vi "IntToBoolean.vi"(1 "Input Int":u8[](array[numeric])) -> (0 "Output Boolean":bool[](array[boolean]))   [LabVIEW 2013]
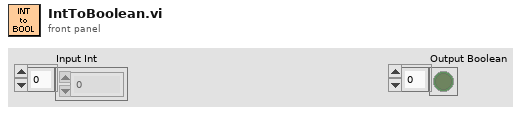
[diagram p1: front panel]
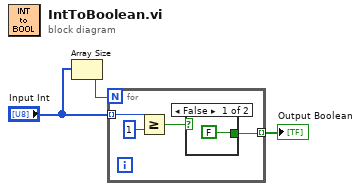
[diagram p0: block diagram]
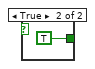
[diagram p2: hidden frame]
diagram:
  n1 = Array Size(array="Input Int") -> (size(s)=w2:i32)
  n2 = for {
    N: w2 -> [_]
    tunnel: "Input Int" -> [w7] mode=indexing
    tunnel: [w4] -> w1 mode=indexing
    n3 = Greater Or Equal?(x=w7, y=u8 1) -> (x >= y?=w5:bool)
    n4 = case shown="False" w5 {
      tunnel: [FALSE TRUE] -> w4
      frame False {
      }
      frame True {
      }
    }
  }
  "Output Boolean" <- w1
